vi "SetForce.vi"(6 "Instance":i32, 8 "error in (no error)":errorcluster, 11 "Cart Force":dbl) -> (0 "error out":errorcluster)   [LabVIEW 2017, in "PendulumLoop.lvlib"]
uses:
  PendulumLoop.lvlib
  Communication/Communication.lvlib
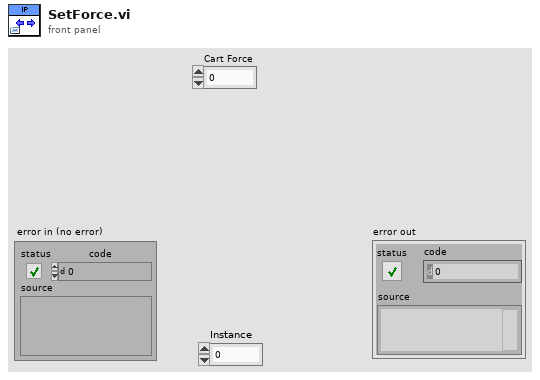
[diagram p1: front panel]
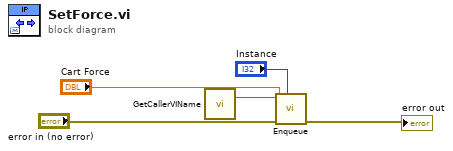
[diagram p0: block diagram]
diagram:
  n1 = call "GetCallerVIName.vi"() -> ("VI name"=w2:string)  [unwired: 11 in]
  n2 = call "Enqueue.vi"("Instance"="Instance", "error in (no error)"="error in (no error)", "Data"="Cart Force", "Msg"=w2) -> ("error out"=→"error out":errorcluster)  [unwired: 7 in]
